vi "Deterine_Warnings.vi"() -> ()   [LabVIEW 2015]
doc: "This simple VI thorws a warning if the Current temp input is greater than the max temp input or less than the min temp input."
panel:
  out "Warning?":bool
  out "Warning Text":string
  in  "Max Temp":dbl=30.0
  in  "Min Temp":dbl=10.0
  in  "Current Temp":dbl=25.0
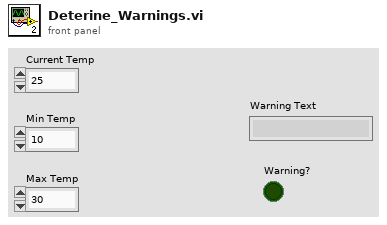
[diagram p1: front panel]
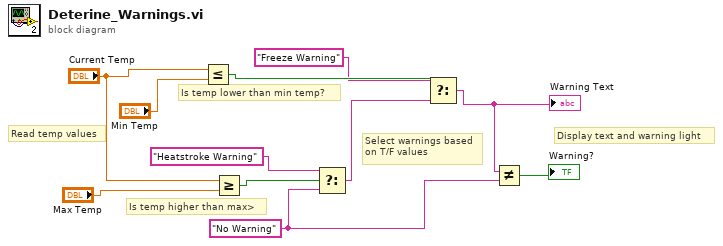
[diagram p0: block diagram]
diagram:
  w3 = "No Warning"
  # "Read temp values"
  # "Display text and warning light"
  # "Select warnings based\non T/F values"
  # "Is temp higher than max>"
  # "Is temp lower than min temp?"
  n1 = Less Or Equal?(x="Current Temp", y="Min Temp") -> (x <= y?=w8:bool)
  n2 = Greater Or Equal?(x="Current Temp", y="Max Temp") -> (x >= y?=w7:bool)
  n3 = Select(t="Heatstroke Warning", s=w7, f=w3) -> (s? t:f=w4:string)
  n4 = Select(t="Freeze Warning", s=w8, f=w4) -> (s? t:f=w2:string)
  "Warning Text" <- w2
  n5 = Not Equal?(x=w2, y=w3) -> (x != y?=→"Warning?":bool)
